vi "Write Number of children.vi"(8 "error in (no error)":errorcluster, 10 "Number of children":i32, 11 "Test Actor in":refnum<class "Example Actor.lvclass">) -> (0 "error out":errorcluster, 3 "Test Actor out":refnum<class "Example Actor.lvclass">)   [LabVIEW 2017, in "Example Actor.lvlib" / "Example Actor.lvclass"]
uses:
  Example Actor.lvclass
  Example Actor.lvclass/Example Actor.ctl
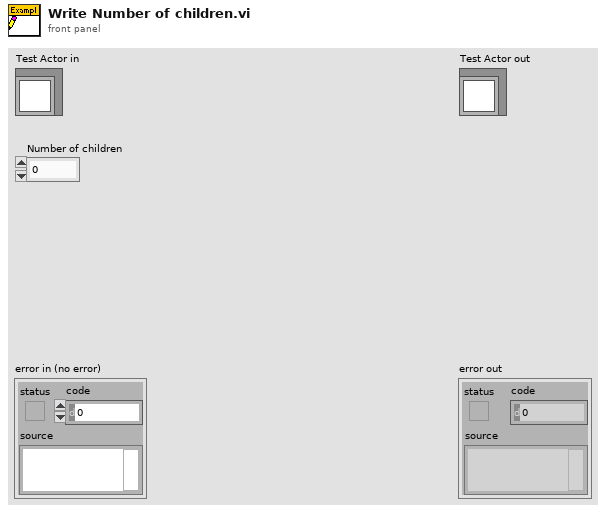
[diagram p1: front panel]
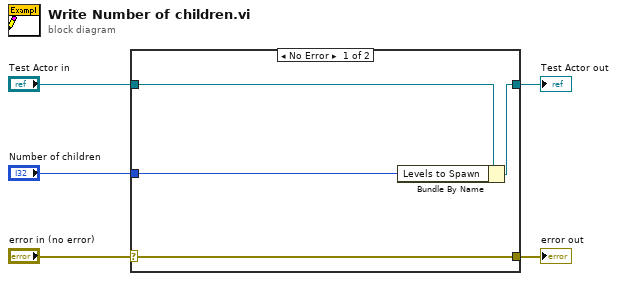
[diagram p0: block diagram]
diagram:
  n1 = case shown="No Error" "error in (no error)" {
    selector: "error in (no error)" -> [w9 w10]
    tunnel: [w9 w10] -> w4
    tunnel: [w7 w11] -> w2
    tunnel: "Test Actor in" -> [w8 w11]
    tunnel: "Number of children" -> [w6 _]
    frame No Error {
      n2 = Bundle By Name(cluster=w8, "Levels to Spawn"=w6) -> (w7:refnum<class "Example Actor.lvclass">)
    }
    frame Error {
    }
  }
  "error out" <- w4
  "Test Actor out" <- w2
